vi "Close SV Connections.vi"(8 "error in (no error)":errorcluster, 11 "SV B-M (Host) in":refnum<class "SV B-M (Host).lvclass">) -> (0 "error out":errorcluster, 3 "SV B-M (Host) out":refnum<class "SV B-M (Host).lvclass">)   [LabVIEW 2015, in "SV B-M (Host).lvclass"]
doc: "Close connections to all open shared variables. Issue a command to the target to do the same and wait on acknowledgement it has been completed."
uses:
  SV B-M (Host).lvclass
  SV B-M (Host).lvclass/SV B-M (Host).ctl
  Listbox - In Progress.vi
  Command & Ack - Send Command.vi
  Command & Ack - Receive Ack.vi
  Process Ack Data - Close SVs.vi
  Listbox - Complete.vi
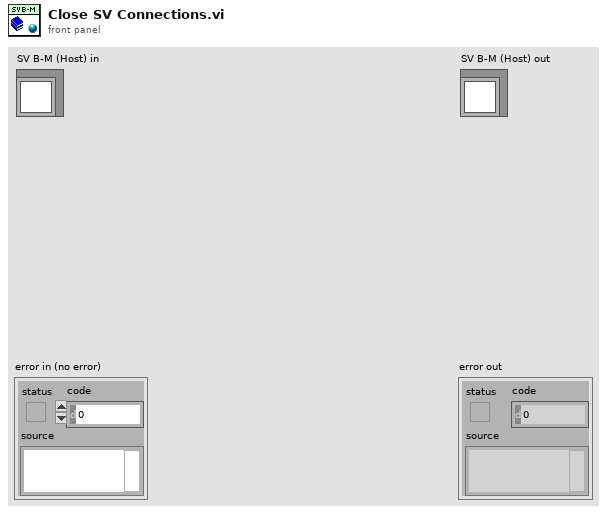
[diagram p1: front panel]
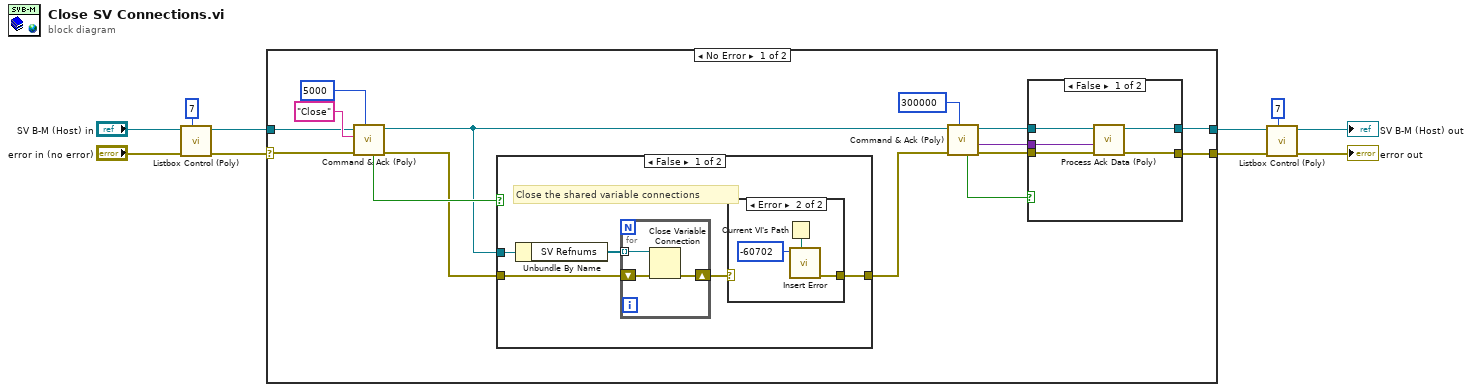
[diagram p0: block diagram]
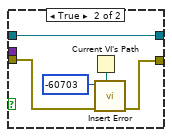
[diagram p2: hidden frame]
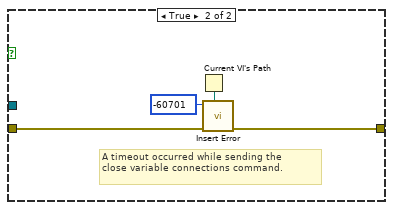
[diagram p4: hidden frame]
diagram:
  n1 = call-poly "Listbox Control (Poly).vi"("Row to Update"=7, "error in (no error)"="error in (no error)", "SV B-M In"="SV B-M (Host) in") -> ("error out"=w7:errorcluster, "SV B-M Out"=w8:refnum<class "SV B-M (Host).lvclass">)  [unwired: 7 in]
  n2 = case shown="No Error" w7 {
    selector: w7 -> [w23 w53]
    tunnel: [w12 w53] -> w3
    tunnel: [w11 w52] -> w4
    tunnel: w8 -> [w22 w52]
    frame No Error {
      n3 = call-poly "Command & Ack (Poly).vi"("Timeout (-1)"=5000, "error in (no error)"=w23, "Message"="Close", "SV B-M (Host) in"=w22) -> ("error out"=w18:errorcluster, "SV B-M (Host) out"=w19:refnum<class "SV B-M (Host).lvclass">, "Timeout?"=w20:bool)  [unwired: 5 in]
      n4 = case shown="False" w20 {
        tunnel: w19 -> [w40 _]
        tunnel: w18 -> [w38 w51]
        tunnel: [w36 w48] -> w17
        frame False {
          # "Close the shared variable connections"
          n5 = Unbundle By Name(w40) -> ("SV Refnums"=w39:refnum<k21>[])
          n6 = for {
            tunnel: w39 -> [w47] mode=indexing
            shift-right: [w45] -> w37
            shift-left: w38 -> [w46]
            n7 = Close Variable Connection(8:w46, 11:w47) -> (0:w45:errorcluster)
          }
          n8 = case shown="Error" w37 {
            selector: w37 -> [w41 _]
            tunnel: [w41 w44] -> w36
            frame No Error {
            }
            frame Error {
              n9 = Current VI's Path() -> (path=w42:path)
              n10 = call "Insert Error.vi"("VI Path"=w42, "Error Code"=-60702) -> ("error out"=w44:errorcluster)  [unwired: 9 in]
            }
          }
        }
        frame True {
          # "A timeout occurred while sending the\nclose variable connections command."
          n11 = Current VI's Path() -> (path=w49:path)
          n12 = call "Insert Error.vi"("VI Path"=w49, "error in (no error)"=w51, "Error Code"=-60701) -> ("error out"=w48:errorcluster)  [unwired: 8 in]
        }
      }
      n13 = call-poly "Command & Ack (Poly).vi"("Timeout (-1)"=300000, "error in (no error)"=w17, "SV B-M (Host) in"=w19) -> ("error out"=w13:errorcluster, "Message Data"=w14:variant, "SV B-M (Host) out"=w15:refnum<class "SV B-M (Host).lvclass">, "Timeout?"=w16:bool)  [unwired: 4 in, 1 out]
      n14 = case shown="False" w16 {
        tunnel: w15 -> [w30 w31]
        tunnel: w14 -> [w29 _]
        tunnel: w13 -> [w28 w35]
        tunnel: [w27 w32] -> w12
        tunnel: [w26 w31] -> w11
        frame False {
          n15 = call-poly "Process Ack Data (Poly).vi"("error in (no error)"=w28, "CPU Load Data"=w29, "SV B-M (Host) in"=w30) -> ("error out"=w27:errorcluster, "SV B-M (Host) out"=w26:refnum<class "SV B-M (Host).lvclass">)  [unwired: 7 in]
        }
        frame True {
          n16 = Current VI's Path() -> (path=w33:path)
          n17 = call "Insert Error.vi"("VI Path"=w33, "error in (no error)"=w35, "Error Code"=-60703) -> ("error out"=w32:errorcluster)  [unwired: 8 in]
        }
      }
    }
    frame Error {
    }
  }
  n18 = call-poly "Listbox Control (Poly).vi"("Row to Update"=7, "error in (no error)"=w3, "SV B-M In"=w4) -> ("error out"=→"error out":errorcluster, "SV B-M Out"=→"SV B-M (Host) out":refnum<class "SV B-M (Host).lvclass">)  [unwired: 7 in]
